vi "Configure Bus Source (I2C).vi"(6 "Data Source (8:Digital Channel 0)":u16(ring)=8 items=["Channel 1", "Channel 2", "Channel 3", "Channel 4", "Math 1", "Math 2", "Math 3", "Math 4", "Digital Channel 0", "Digital Channel 1", "Digital Channel 2", "Digital Channel 3", "Digital Channel 4", "Digital Channel 5", "Digital Channel 6", "Digital Channel 7", "Digital Channel 8", "Digital Channel 9", "Digital Channel 10", "Digital Channel 11", "Digital Channel 12", "Digital Channel 13", "Digital Channel 14", "Digital Channel 15"], 7 "Clock Source (9:Digital Channel 1)":u16(ring)=9 items=["Channel 1", "Channel 2", "Channel 3", "Channel 4", "Math 1", "Math 2", "Math 3", "Math 4", "Digital Channel 0", "Digital Channel 1", "Digital Channel 2", "Digital Channel 3", "Digital Channel 4", "Digital Channel 5", "Digital Channel 6", "Digital Channel 7", "Digital Channel 8", "Digital Channel 9", "Digital Channel 10", "Digital Channel 11", "Digital Channel 12", "Digital Channel 13", "Digital Channel 14", "Digital Channel 15"], 8 "error in (no error)":errorcluster, 9 "Enable R/W Inclusion In Address(F:Disable)":bool, 10 "BUS Number (0:Bus 1)":u8(ring) items=["Bus 1", "Bus 2", "Bus 3", "Bus 4", "Bus 5", "Bus 6", "Bus 7", "Bus 8", "Bus 9", "Bus 10", "Bus 11", "Bus 12", "Bus 13", "Bus 14", "Bus 15", "Bus 16"], 11 "VISA resource name":refnum<visa-resource-name>) -> (0 "error out":errorcluster, 3 "VISA resource name out":refnum<visa-resource-name>)   [LabVIEW 2015, in "Tektronix 7000 Series.lvlib"]
doc: "Configures I2C Bus Setting for an oscilloscope.\n\n<B>Note:</B> \nThese commands are not supported by TDS or CSA models."
uses:
  <instrlib>/Tektronix 7000 Series/Tektronix 7000 Series.lvlib
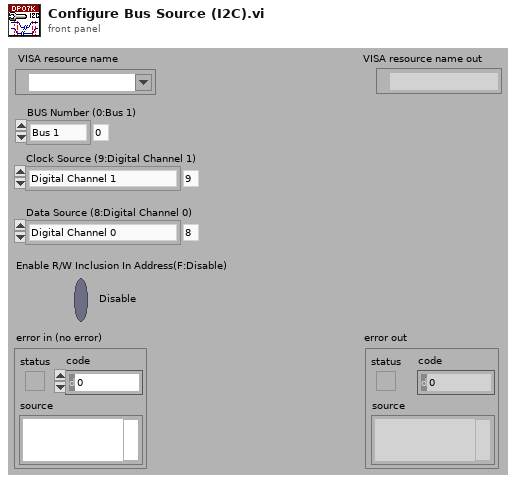
[diagram p1: front panel]
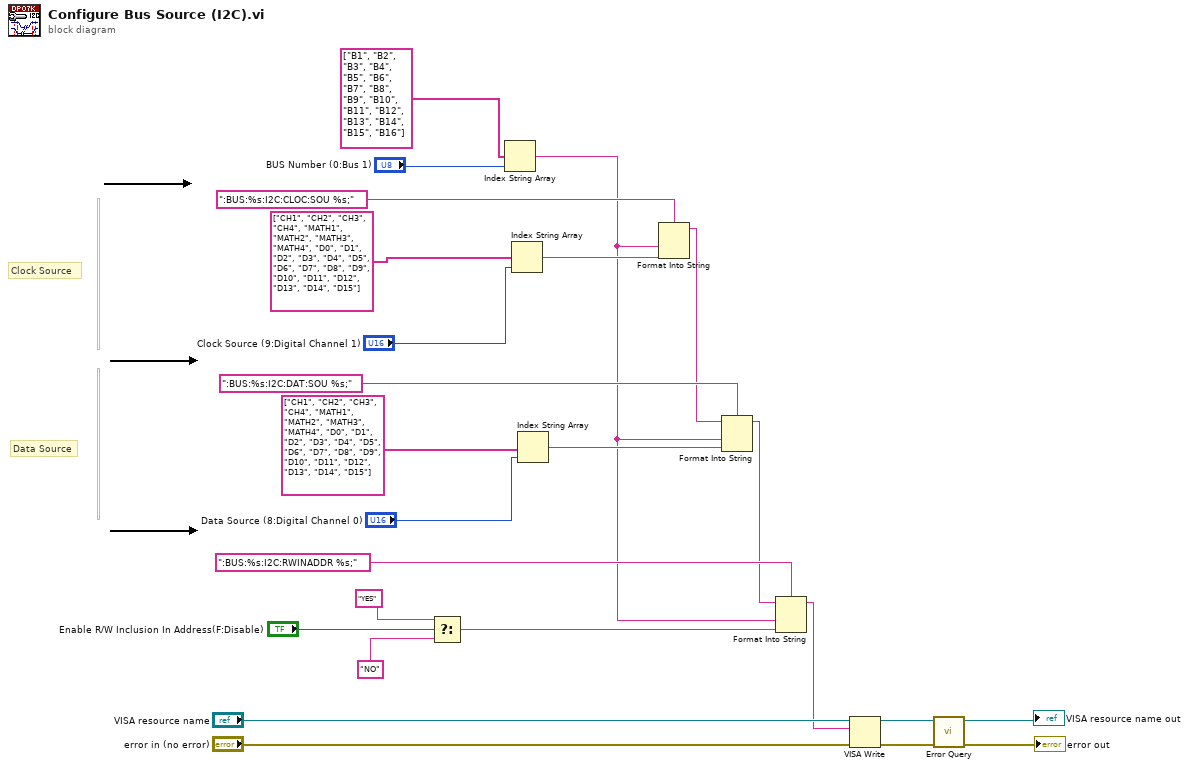
[diagram p0: block diagram]
diagram:
  # "Data Source"
  # "Clock Source"
  n1 = Select(t="YES", s="Enable R/W Inclusion In Address(F:Disable)", f="NO") -> (s? t:f=w15:string)
  n2 = Index String Array(1:"BUS Number (0:Bus 1)", 2:string[] ["B1", "B2", "B3", "B4", "B5", "B6", "B7", "B8", "B9", "B10", "B11", "B12", "B13", "B14", "B15", "B16"]) -> (0:w8:string)  [unwired: 1 out]
  n3 = Index String Array(1:"Clock Source (9:Digital Channel 1)", 2:string[] ["CH1", "CH2", "CH3", "CH4", "MATH1", "MATH2", "MATH3", "MATH4", "D0", "D1", "D2", "D3", "D4", "D5", "D6", "D7", "D8", "D9", "D10", "D11", "D12", "D13", "D14", "D15"]) -> (0:w13:string)  [unwired: 1 out]
  n4 = Index String Array(1:"Data Source (8:Digital Channel 0)", 2:string[] ["CH1", "CH2", "CH3", "CH4", "MATH1", "MATH2", "MATH3", "MATH4", "D0", "D1", "D2", "D3", "D4", "D5", "D6", "D7", "D8", "D9", "D10", "D11", "D12", "D13", "D14", "D15"]) -> (0:w10:string)  [unwired: 1 out]
  n5 = Format Into String(format string=":BUS:%s:I2C:CLOC:SOU %s;", w8, w13) -> (resulting string=w11:string)  [unwired: 2 in, 1 out]
  n6 = Format Into String(format string=":BUS:%s:I2C:DAT:SOU %s;", initial string=w11, w8, w10) -> (resulting string=w6:string)  [unwired: 1 in, 1 out]
  n7 = Format Into String(format string=":BUS:%s:I2C:RWINADDR %s;", initial string=w6, w8, w15) -> (resulting string=w7:string)  [unwired: 1 in, 1 out]
  n8 = VISA Write(VISA resource name="VISA resource name", write buffer=w7, error in (no error)="error in (no error)") -> (VISA resource name out=w21:refnum<visa-resource-name>, error out=w20:errorcluster)  [unwired: 1 out]
  n9 = call <instrlib>:"Error Query.vi"("error in (no error)"=w20, "VISA resource name"=w21) -> ("error out"=→"error out":errorcluster, "VISA resource name out"=→"VISA resource name out":refnum<visa-resource-name>)  [unwired: 8 out]
